vi "DCA Convert 1.6 - 1.7 to 1.8.vi"(1 "DCA 1.6 - 1.7 Test Parameters":T2={"Tag"="", "Use Instrument"=FALSE, "Quick Mode"=FALSE, "Topology"=enum."Pi", "Zo"=50.0, "Range"=0, "Resolution"=0, "Blank Screen"=FALSE, "Limits"=[], "Reports"={"Reports to Generate"=[], "Print Reports"=TRUE}, "Lock Topology"=FALSE, "Normalize"=TRUE, "ATTN Calc"=enum."Power"} {"Resolution" items=["Auto", "4 1/2", "5 1/2", "6 1/2"]; "Range" items=["Auto", "Min", "Max", "100", "1,000", "10,000", "100,000", "1,000,000", "10,000,000", "100,000,000"]; "Limits"."Run" min=1 step=1}) -> (0 "DCA 1.8 Test Parameters":T1={"Tag"="", "Use Instrument"=FALSE, "Quick Mode"=FALSE, "Topology"=enum."Pi", "Zo"=50.0, "Range"=0, "Resolution"=0, "Blank Screen"=FALSE, "Limits"=[], "Datasheets"={"Datasheets to Generate"=[], "Print Datasheets"=TRUE}, "Lock Topology"=FALSE, "Normalize"=TRUE, "ATTN Calc"=enum."Power"} {"Resolution" items=["Auto", "4 1/2", "5 1/2", "6 1/2"]; "Range" items=["Auto", "Min", "Max", "100", "1,000", "10,000", "100,000", "1,000,000", "10,000,000", "100,000,000"]; "Limits"."Run" min=1 step=1})   [LabVIEW 2011]
uses:
  TypeDefs/DCA Test Parameters v1.6-1.7.ctl
  TypeDefs/DCA Test Parameters v1.8.ctl
panel:
  # "="
  # "="
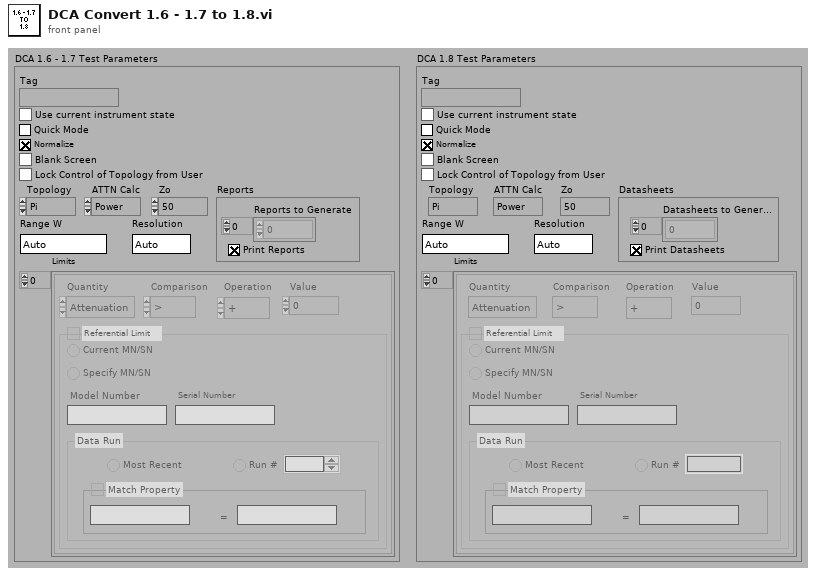
[diagram p1: front panel]
types:
  T1 = typedef "DCA Test Parameters v1.8.ctl" = cluster{"Tag":string, "Use Instrument":bool, "Quick Mode":bool, "Topology":enum32{"Pi", "T"}, "Zo":dbl, "Range":u16, "Resolution":u16, "Blank Screen":bool, "Limits":cluster{"Quantity":enum16{"Attenuation", "Zin", "Zout", "R1", "R2", "R3", "Rab", "Rac", "Rbc"}, "Comparison":enum16{">", ">=", "<", "<=", "+", "-"}, "Operation":enum16{"+", "-"}, "Value":dbl, "Ref Limit":bool, "Ref Type":enum32{"Current", "Specify"}, "Model":string, "Serial":string, "Run Type":enum32{"Most Recent", "Run #"}, "Run":i32, "Match Property":bool, "Property":string, "Property Value":string}[], "Datasheets":cluster{"Datasheets to Generate":i32[], "Print Datasheets":bool}, "Lock Topology":bool, "Normalize":bool, "ATTN Calc":enum32{"Power", "Voltage"}}
  T2 = typedef "DCA Test Parameters v1.6-1.7.ctl" = cluster{"Tag":string, "Use Instrument":bool, "Quick Mode":bool, "Topology":enum32{"Pi", "T"}, "Zo":dbl, "Range":u16, "Resolution":u16, "Blank Screen":bool, "Limits":cluster{"Quantity":enum16{"Attenuation", "Zin", "Zout", "R1", "R2", "R3", "Rab", "Rac", "Rbc"}, "Comparison":enum16{">", ">=", "<", "<=", "+", "-"}, "Operation":enum16{"+", "-"}, "Value":dbl, "Ref Limit":bool, "Ref Type":enum32{"Current", "Specify"}, "Model":string, "Serial":string, "Run Type":enum32{"Most Recent", "Run #"}, "Run":i32, "Match Property":bool, "Property":string, "Property Value":string}[], "Reports":cluster{"Reports to Generate":i32[], "Print Reports":bool}, "Lock Topology":bool, "Normalize":bool, "ATTN Calc":enum32{"Power", "Voltage"}}
  T3 = cluster{"Quantity":enum16{"Attenuation", "Zin", "Zout", "R1", "R2", "R3", "Rab", "Rac", "Rbc"}, "Comparison":enum16{">", ">=", "<", "<=", "+", "-"}, "Operation":enum16{"+", "-"}, "Value":dbl, "Ref Limit":bool, "Ref Type":enum32{"Current", "Specify"}, "Model":string, "Serial":string, "Run Type":enum32{"Most Recent", "Run #"}, "Run":i32, "Match Property":bool, "Property":string, "Property Value":string}[]
  T4 = cluster{"Reports to Generate":i32[], "Print Reports":bool}
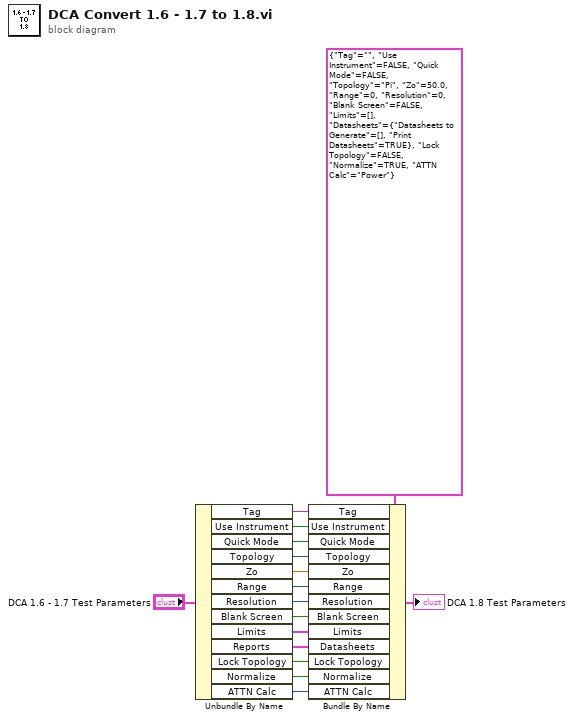
[diagram p0: block diagram]
diagram:
  n1 = Unbundle By Name("DCA 1.6 - 1.7 Test Parameters") -> ("Tag"=w4:string, "Use Instrument"=w5:bool, "Quick Mode"=w6:bool, "Topology"=w7:enum32{"Pi", "T"}, "Zo"=w8:dbl, "Range"=w9:u16, "Resolution"=w10:u16, "Blank Screen"=w11:bool, "Limits"=w12:T3, "Reports"=w13:T4, "Lock Topology"=w14:bool, "Normalize"=w15:bool, "ATTN Calc"=w16:enum32{"Power", "Voltage"})
  n2 = Bundle By Name(cluster=T1 {"Tag"="", "Use Instrument"=FALSE, "Quick Mode"=FALSE, "Topology"=enum."Pi", "Zo"=50.0, "Range"=0, "Resolution"=0, "Blank Screen"=FALSE, "Limits"=[], "Datasheets"={"Datasheets to Generate"=[], "Print Datasheets"=TRUE}, "Lock Topology"=FALSE, "Normalize"=TRUE, "ATTN Calc"=enum."Power"} ("DCA 1.9 Test Parameters"), "Tag"=w4, "Use Instrument"=w5, "Quick Mode"=w6, "Topology"=w7, "Zo"=w8, "Range"=w9, "Resolution"=w10, "Blank Screen"=w11, "Limits"=w12, "Datasheets"=w13, "Lock Topology"=w14, "Normalize"=w15, "ATTN Calc"=w16) -> (→"DCA 1.8 Test Parameters":T1)
